vi "TDMS-Datei laden.vi"(11 "Dateipfad":path) -> (0 "Datentypen":string[](array[string]), 1 "Namen":string[](array[string]), 2 "Zuordnungstabelle":i16[][](array[numeric]), 3 "Programm":T1[](array[typedef]), 4 "Eigenschaften":T3, 5 "Fixbild (Pixmap)":u32[][](array[numeric]), 7 "Fixbild":T1[](array[typedef]))   [LabVIEW 2020, in "Anlagenuebersicht.lvlib" / "VisBx Anzeige.lvlib" / "TDMS laden.lvlib"]
doc: "Öffnet eine TDMS-Datei für die Visualisierungs-Anwendung \"VisBx Anzeige\" und stellt alle für die Visualisierung benötigten Daten bereit:\n\nFixbild: \nWird nur für Editieren (VisBx-Editor) gebraucht, enthält alle Einzelschritte zum Aufbau eines Fixbildes.\n\nFixbild (Pixmap):\nEnthält das fertige Fixbild in kompakter Form um den Bildaufbau zu beschleunigen.\n\nProgramm:\nBesteht aus Programmschritten mit Zeichenbefehlen und Daten für den Aufbau eines bewegten Bildes.\n\nZuordnungstabelle:\nStellt die Verbindung zwischen dem aktuellen Prozesszustand und den zugehörigen Zeichenbefehlen in \"Programm\" her.\n\nNamen:\nNamen aller Prozessvariablen, die Grundlage für die TDMS-Datei waren.\n\nDatentypen:\nDatentypen aller Prozessvariablen.\n\nEigenschaften:\nCluster mit den Elementen\n Größe: Bildgröße der Visualisierung (Width, Height)\n URL: String mit URL der XML-Umgebungsvariablen für die Prozesskopplung\n Raster: letztes Rastermaß (wird nur für Editor gebraucht)\n Hintergrund: Hintergrundfarbe der Visualisierung (nur für Editor)."
uses:
  TDMS laden.lvlib
  VisParameter/VisSchritt.ctl
  VisParameter/VisSchritt-Typ.ctl
  TDMS-Eigenschaften.ctl
  <vilib>/Utility/miscctls.llb/LVBoundsTypeDef.ctl
  VisParameter/VisParam-Typdef.lvlib
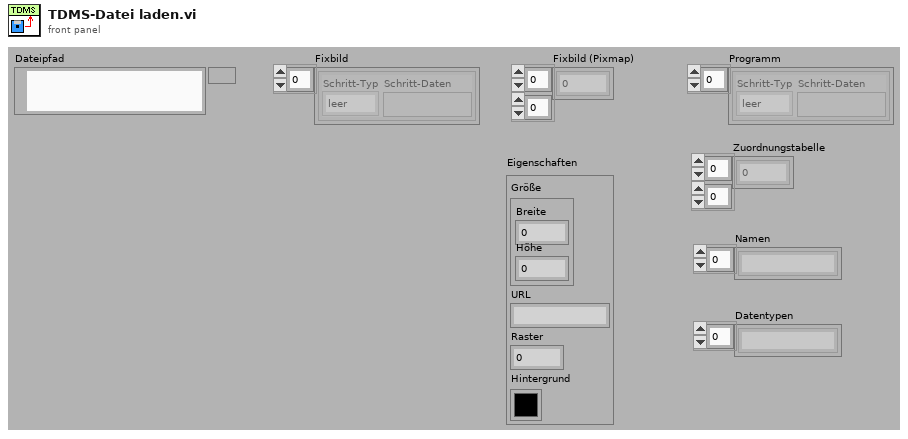
[diagram p1: front panel]
types:
  T1 = typedef "VisParam-Typdef.lvlib/VisSchritt.ctl" = cluster{"Schritt-Typ":T2, "Schritt-Daten":variant}
  T2 = typedef "VisParam-Typdef.lvlib/VisSchritt-Typ.ctl" = enum16{"leer", "Punkt", "Linie", "Linienzug", "Fixtext", "Textrechteck", "Ziffernanzeige", "Rechteck", "Rechteck rund", "Ellipse", "Bogen", "Kreis", "Pixmap"}
  T3 = typedef "Anlagenuebersicht.lvlib/VisBx Anzeige.lvlib/TDMS laden.lvlib/TDMS-Eigenschaften.ctl" = cluster{"Größe":T4, "URL":string, "Raster":i16, "Hintergrund":u32}
  T4 = typedef "LVBoundsTypeDef.ctl" = cluster{"Width":u32, "Height":u32}
  T5 = enum16{"open", "open or create", "create or replace", "create", "open (read-only)"}
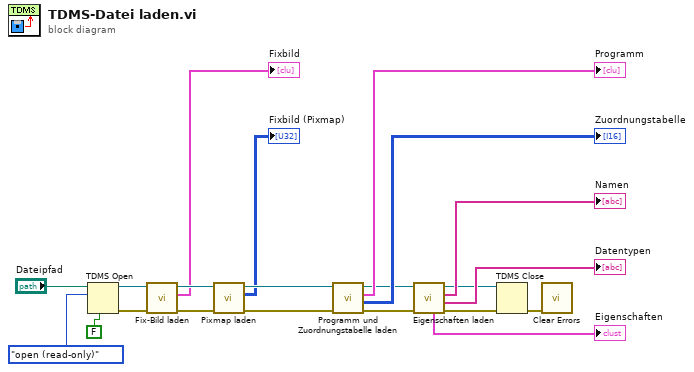
[diagram p0: block diagram]
diagram:
  n1 = TDMS Open(6:FALSE ("Pufferung deaktivieren (T)"), 10:T5."open (read-only)" ("Operation (0:Öffnen)"), 11:"Dateipfad") -> (0:w4:errorcluster, 3:w6:refnum<k34>)  [unwired: 4 in]
  n2 = call "Fix-Bild laden.vi"("error in (no error)"=w4, "TDMS-Datei"=w6) -> ("error out"=w3:errorcluster, "Fixbild"=→"Fixbild":T1[], "TDMS-Datei (Ausgang)"=w5:refnum<k34>)  [unwired: 7 in]
  n3 = call "Pixmap laden.vi"("error in (no error)"=w3, "TDMS-Datei"=w5) -> ("error out"=w9:errorcluster, "Pixmap"=→"Fixbild (Pixmap)":u32[][], "TDMS-Datei (Ausgang)"=w8:refnum<k34>)  [unwired: 7 in]
  n4 = call "Programm und Zuordnungstabelle laden.vi"("error in (no error)"=w9, "TDMS-Datei"=w8) -> ("error out"=w14:errorcluster, "Zuordnungstabelle"=→"Zuordnungstabelle":i16[][], "Programm"=→"Programm":T1[], "TDMS-Datei (Ausgang)"=w15:refnum<k34>)  [unwired: 6 out]
  n5 = call "Eigenschaften laden.vi"("error in (no error)"=w14, "TDMS-Datei"=w15) -> ("error out"=w12:errorcluster, "Datentypen"=→"Datentypen":string[], "Namen"=→"Namen":string[], "TDMS-Datei (Ausgang)"=w13:refnum<k34>, "Eigenschaften"=→"Eigenschaften":T3)  [unwired: 1 in, 4 out]
  n6 = TDMS Close(8:w12, 11:w13) -> (0:w1:errorcluster)  [unwired: 1 out]
  n7 = call <vilib>:"Clear Errors.vi"("error in (no error)"=w1) -> ()  [unwired: 5 in, 2 out]
